vi "Wiimote Enable IR Sensor.vi"(8 "error in":errorcluster, 11 "hWiimoteHandle in":u32 format="%08x") -> (0 "error out":errorcluster, 3 "hWiimoteHandle out":u32 format="%08x")   [LabVIEW 2012, in "Wiimote.lvlib"]
uses:
  Wiimote.lvlib
  Wiimote Address Space.ctl
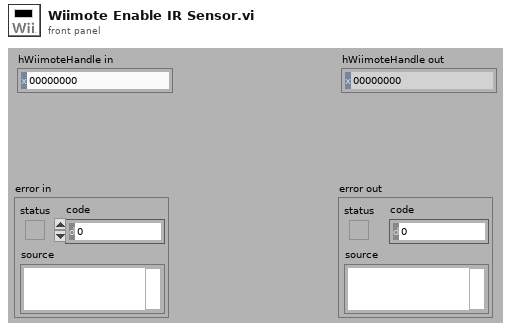
[diagram p1: front panel]
types:
  T1 = typedef "Wiimote.lvlib/Wiimote Address Space.ctl" = u8
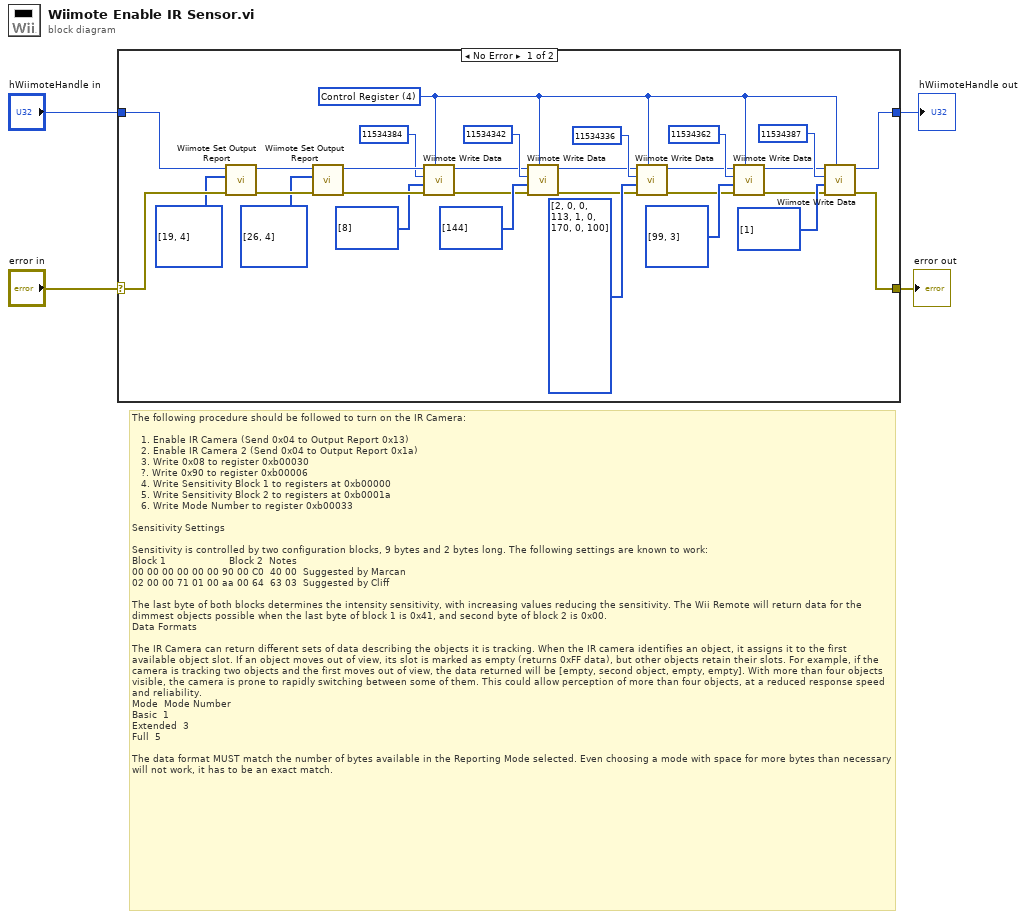
[diagram p0: block diagram]
diagram:
  # "The following procedure should be followed to turn on the IR Camera:\n\n   1. Enable IR Camera (Send 0x04 to Output Report 0x13)\n   2. Enable IR Camera 2 (Send 0x04 to Output Report 0x1a)\n   3. Write 0x08 to register 0xb00030\n   ?. Write 0x90 to register 0xb00006\n   4. Write Sensitivity Block 1 to registers at 0xb00000\n   5. Write Sensitivity Block 2 to registers at 0xb0001a\n   6. Write Mode Number to register 0xb00033 \n\nSensitivity Settings\n\nSensitivity is controlled by two configuration blocks, 9 bytes and 2 bytes long. The following settings are known to work:\nBlock 1 \t                   Block 2 \tNotes\n00 00 00 00 00 00 90 00 C0 \t40 00 \tSuggested by Marcan\n02 00 00 71 01 00 aa 00 64 \t63 03 \tSuggested by Cliff\n\nThe last byte of both blocks determines the intensity sensitivity, with increasing values reducing the sensitivity. The Wii Remote will return data for the dimmest objects possible when the last byte of block 1 is 0x41, and second byte of block 2 is 0x00.\nData Formats\n\nThe IR Camera can return different sets of data describing the objects it is tracking. When the IR camera identifies an object, it assigns it to the first available object slot. If an object moves out of view, its slot is marked as empty (returns 0xFF data), but other objects retain their slots. For example, if the camera is tracking two objects and the first moves out of view, the data returned will be [empty, second object, empty, empty]. With more than four objects visible, the camera is prone to rapidly switching between some of them. This could allow perception of more than four objects, at a reduced response speed and reliability.\nMode \tMode Number\nBasic \t1\nExtended \t3\nFull \t5\n\nThe data format MUST match the number of bytes available in the Reporting Mode selected. Even choosing a mode with space for more bytes than necessary will not work, it has to be an exact match."
  n1 = case shown="No Error" "error in" {
    selector: "error in" -> [w31 w35]
    tunnel: [w6 w35] -> w3
    tunnel: "hWiimoteHandle in" -> [w33 w34]
    tunnel: [w7 w34] -> w1
    frame No Error {
      w5 = T1 4 items=["EEPROM Memory"=0, "Control Register"=4] ("Address Space")
      n2 = call "Wiimote Set Output Report.vi"("error in"=w31, "pReportBuffer in"=u8[] [19, 4] ("appended array"), "hWiimoteHandle in"=w33) -> ("error out"=w30:errorcluster, "hWiimoteHandle out"=w32:u32)  [unwired: 7 in]
      n3 = call "Wiimote Set Output Report.vi"("error in"=w30, "pReportBuffer in"=u8[] [26, 4] ("appended array"), "hWiimoteHandle in"=w32) -> ("error out"=w26:errorcluster, "hWiimoteHandle out"=w27:u32)  [unwired: 7 in]
      n4 = call "Wiimote Write Data.vi"("Address Space"=w5, "error in"=w26, "pReportBuffer in"=u8[] [8], "Offset"=u32 11534384, "hWiimoteHandle in"=w27) -> ("error out"=w20:errorcluster, "hWiimoteHandle out"=w21:u32)  [unwired: 5 in]
      n5 = call "Wiimote Write Data.vi"("Address Space"=w5, "error in"=w20, "pReportBuffer in"=u8[] [144], "Offset"=u32 11534342, "hWiimoteHandle in"=w21) -> ("error out"=w16:errorcluster, "hWiimoteHandle out"=w17:u32)  [unwired: 5 in]
      n6 = call "Wiimote Write Data.vi"("Address Space"=w5, "error in"=w16, "pReportBuffer in"=u8[] [2, 0, 0, 113, 1, 0, 170, 0, 100], "Offset"=u32 11534336, "hWiimoteHandle in"=w17) -> ("error out"=w12:errorcluster, "hWiimoteHandle out"=w13:u32)  [unwired: 5 in]
      n7 = call "Wiimote Write Data.vi"("Address Space"=w5, "error in"=w12, "pReportBuffer in"=u8[] [99, 3], "Offset"=u32 11534362, "hWiimoteHandle in"=w13) -> ("error out"=w8:errorcluster, "hWiimoteHandle out"=w9:u32)  [unwired: 5 in]
      n8 = call "Wiimote Write Data.vi"("Address Space"=w5, "error in"=w8, "pReportBuffer in"=u8[] [1], "Offset"=u32 11534387, "hWiimoteHandle in"=w9) -> ("error out"=w6:errorcluster, "hWiimoteHandle out"=w7:u32)  [unwired: 5 in]
    }
    frame Error {
    }
  }
  "error out" <- w3
  "hWiimoteHandle out" <- w1
